vi "Calibrate Path Group.vi"(7 "Path":path=path "C:/G0X/Data", 8 "error in (no error)":errorcluster, 10 "Module":i32(ring)=1 items=["Master"=1, "Slave"=2]) -> (0 "error out":errorcluster)   [LabVIEW 2009, in "POLARIS BME DG.lvlib"]
doc: "long CalibratePathGroup(int* p_module, char* Path);"
uses:
  POLARIS BME DG.lvlib
  BME DLL/DelayGenerator.dll
panel:
  # "NOTICE -- YOU MUST LEAVE THIS NOTICE IN PLACE.  PER THE TERMS OF THE LICENSE BELOW, YOU MAY SUBLICENSE THIS SOFTWARE \nIN ANY WAY THAT DOES NOT CONFLICT WITH THIS LICENSE.\n\n### BSD License (http://www.opensource.org/licenses/bsd-license.php) Begin ###\n \nCopyright (c) 2011, Applied Energetics, http://www.appliedenergetics.com,\n                               Richard Schwerdtfeger, <rschwerdtfeger@appliedenergetics.com>\n\nAll rights reserved.\n\nRedistribution and use in source and binary forms, with or without modification, are permitted provided that the \nfollowing conditions are met:\n\n    * Redistributions of source code must retain the above copyright notice, this list of conditions and the following disclaimer.\n    * Redistributions in binary form must reproduce the above copyright notice, this list of conditions and the following disclaimer \n       in the documentation and/or other materials provided with the distribution.\n    * Neither the name of Richard Schwerdtfeger, Applied Energetics, Inc., nor the names of its contributors may be used to \n       endorse or promote products derived from this software without specific prior written permission.\n\nTHIS SOFTWARE IS PROVIDED BY THE COPYRIGHT HOLDERS AND CONTRIBUTORS \"AS IS\" AND ANY EXPRESS OR IMPLIED WARRANTIES, \nINCLUDING, BUT NOT LIMITED TO, THE IMPLIED WARRANTIES OF MERCHANTABILITY AND FITNESS FOR A PARTICULAR PURPOSE ARE \nDISCLAIMED. IN NO EVENT SHALL THE COPYRIGHT OWNER OR CONTRIBUTORS BE LIABLE FOR ANY DIRECT, INDIRECT, INCIDENTAL,\n SPECIAL, EXEMPLARY, OR CONSEQUENTIAL DAMAGES (INCLUDING, BUT NOT LIMITED TO, PROCUREMENT OF SUBSTITUTE GOODS OR \nSERVICES; LOSS OF USE, DATA, OR PROFITS; OR BUSINESS INTERRUPTION) HOWEVER CAUSED AND ON ANY THEORY OF LIABILITY, \nWHETHER IN CONTRACT, STRICT LIABILITY, OR TORT (INCLUDING NEGLIGENCE OR OTHERWISE) ARISING IN ANY WAY OUT OF THE USE \nOF THIS SOFTWARE, EVEN IF ADVISED OF THE POSSIBILITY OF SUCH DAMAGE.\n\n### BSD License End ###"
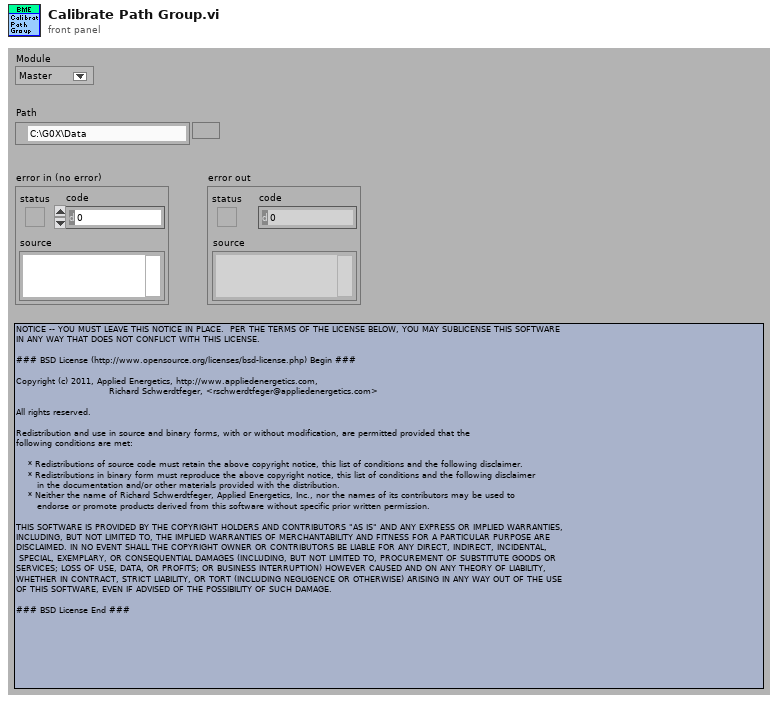
[diagram p1: front panel]
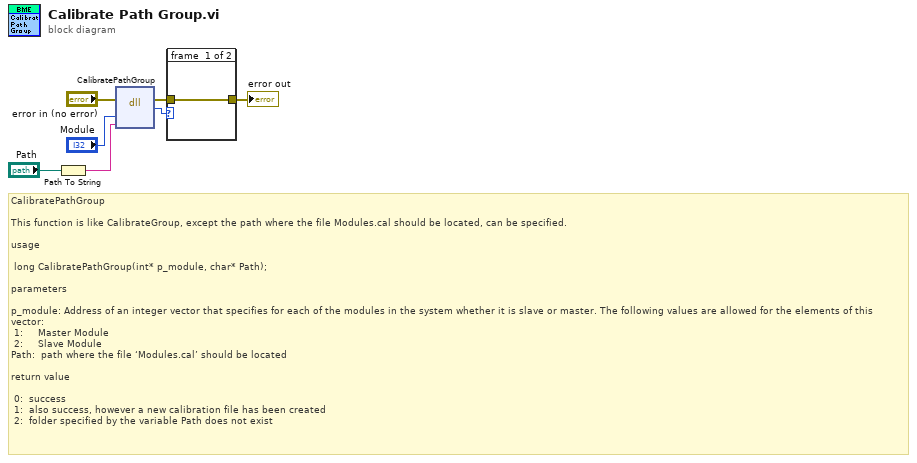
[diagram p0: block diagram]
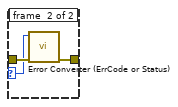
[diagram p2: hidden frame]
diagram:
  # "CalibratePathGroup\n\nThis function is like CalibrateGroup, except the path where the file Modules.cal should be located, can be specified.\n\nusage\n\n\tlong CalibratePathGroup(int* p_module, char* Path);\n\nparameters\n\np_module:\tAddress of an integer vector that specifies for each of the modules in the system whether it is slave or master. The following values are allowed for the elements of this vector:\n\t1:     Master Module\n\t2:     Slave Module\nPath:\t\tpath where the file ‘Modules.cal’ should be located\n\nreturn value\n\n\t0:  success\n\t1:  also success, however a new calibration file has been created\n\t2:  folder specified by the variable Path does not exist"
  n1 = Path To String(path="Path") -> (string=w2:string)
  n2 = dll-call lib="C:/CS Framework/LVSCC/LV2009/GPL/Projects/cs-framework/CSClass/CSPOLARIS/POLARIS BME DG/BME DLL/DelayGenerator.*" fn="CalibratePathGroup"(error in="error in (no error)", "p_module"="Module", "Path"=w2) -> (error out=w5:errorcluster, w1:i32)  [unwired: 4 in, 1 out]
  n3 = case shown="Default" w1 {
    selector: w1 -> [_ w9]
    tunnel: w5 -> [w8 w11]
    tunnel: [w8 w10] -> w4
    frame #0 {
    }
    frame #1 {
      n4 = call "Error Converter (ErrCode or Status).vi"("error in (no error)"=w11, "error code"=w9) -> ("error out"=w10:errorcluster)  [unwired: 9 out]
    }
  }
  "error out" <- w4
